vi "detect chassis modules.vi"(8 "error in":errorcluster, 11 "Controller in":refnum<class "Controller.lvclass">=refnum) -> (0 "error out":errorcluster, 3 "Controller out":refnum<class "Controller.lvclass">)   [LabVIEW 2013, in "SMI.lvlib" / "Chassis.lvclass"]
uses:
  Chassis.lvclass
  C Series Module/C Series Module.lvclass
  PXI Module/PXI Module.lvclass
  Controller/Controller.lvclass
  Device/Device.lvclass
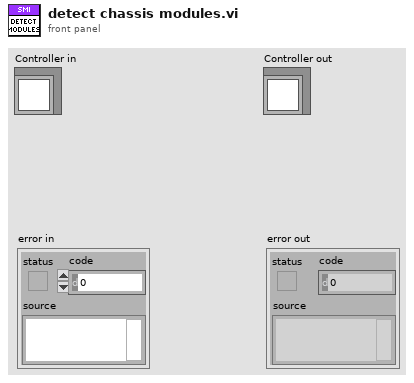
[diagram p1: front panel]
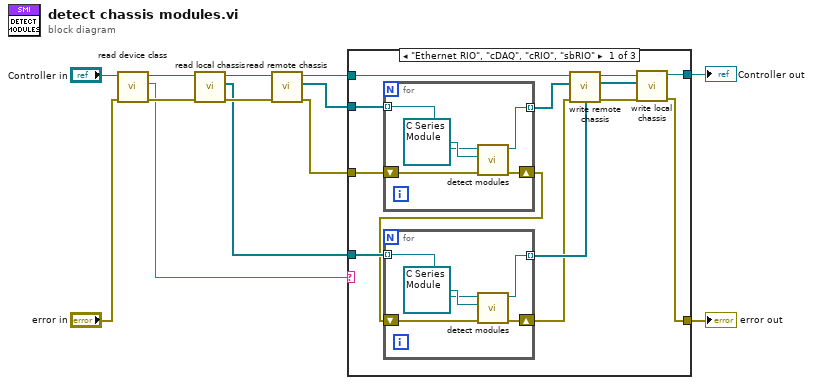
[diagram p0: block diagram]
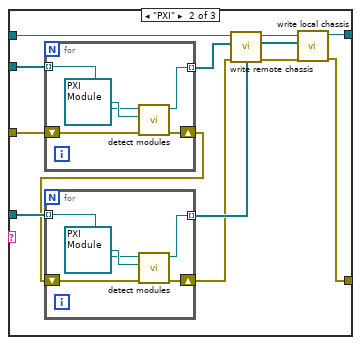
[diagram p2: hidden frame]
diagram:
  n1 = call-dynamic "read device class.vi"("error in"="error in", "device in"="Controller in") -> ("error out"=w9:errorcluster, "device class"=w1:string, "device out"=w2:refnum<class "Device.lvclass">)  [unwired: 7 in]
  n2 = call-dynamic "read local chassis.vi"("error in (no error)"=w9, "Controller in"=w2) -> ("error out"=w4:errorcluster, "local chassis"=w3:refnum<class "Chassis.lvclass">[], "Controller out"=w10:refnum<class "Controller.lvclass">)  [unwired: 7 in]
  n3 = call-dynamic "read remote chassis.vi"("error in (no error)"=w4, "Controller in"=w10) -> ("error out"=w8:errorcluster, "remote chassis"=w6:refnum<class "Chassis.lvclass">[], "Controller out"=w7:refnum<class "Controller.lvclass">)  [unwired: 7 in]
  n4 = case shown="\"Ethernet RIO\", \"cDAQ\", \"cRIO\", \"sbRIO\"" w1 {
    tunnel: [w14 w36 w59] -> w11
    tunnel: w8 -> [w18 w40 w59]
    tunnel: w3 -> [w25 w47 _]
    tunnel: w6 -> [w24 w46 _]
    tunnel: w7 -> [w23 w45 w58]
    tunnel: [w21 w43 w58] -> w5
    frame "Ethernet RIO", "cDAQ", "cRIO", "sbRIO" {
      n5 = for {
        tunnel: w24 -> [w29] mode=indexing
        tunnel: [w28] -> w20 mode=indexing
        shift-right: [w27] -> w17
        shift-left: w18 -> [w26]
        n6 = call-dynamic "detect modules.vi"("error in"=w26, "Module in"=refnum<class "C Series Module.lvclass"> refnum ("SMI.lvlib:C Series Module.lvclass"), "Chassis in"=w29) -> ("error out"=w27:errorcluster, "Chassis out"=w28:refnum<class "Chassis.lvclass">)  [unwired: 6 in, 1 out]
      }
      n7 = for {
        tunnel: w25 -> [w34] mode=indexing
        tunnel: [w33] -> w19 mode=indexing
        shift-right: [w32] -> w15
        shift-left: w17 -> [w31]
        n8 = call-dynamic "detect modules.vi"("error in"=w31, "Module in"=refnum<class "C Series Module.lvclass"> refnum ("SMI.lvlib:C Series Module.lvclass"), "Chassis in"=w34) -> ("error out"=w32:errorcluster, "Chassis out"=w33:refnum<class "Chassis.lvclass">)  [unwired: 6 in, 1 out]
      }
      n9 = call-dynamic "write remote chassis.vi"("error in (no error)"=w15, "remote chassis"=w20, "Controller in"=w23) -> ("error out"=w16:errorcluster, "Controller out"=w22:refnum<class "Controller.lvclass">)  [unwired: 7 in]
      n10 = call-dynamic "write local chassis.vi"("error in (no error)"=w16, "local chassis"=w19, "Controller in"=w22) -> ("error out"=w14:errorcluster, "Controller out"=w21:refnum<class "Controller.lvclass">)  [unwired: 7 in]
    }
    frame "PXI" {
      n11 = for {
        tunnel: w46 -> [w51] mode=indexing
        tunnel: [w50] -> w42 mode=indexing
        shift-right: [w49] -> w39
        shift-left: w40 -> [w48]
        n12 = call-dynamic "detect modules.vi"("error in"=w48, "PXI Module in"=refnum<class "PXI Module.lvclass"> refnum ("SMI.lvlib:PXI Module.lvclass"), "Chassis in"=w51) -> ("error out"=w49:errorcluster, "Chassis out"=w50:refnum<class "Chassis.lvclass">)  [unwired: 6 in, 1 out]
      }
      n13 = for {
        tunnel: w47 -> [w56] mode=indexing
        tunnel: [w55] -> w41 mode=indexing
        shift-right: [w54] -> w37
        shift-left: w39 -> [w53]
        n14 = call-dynamic "detect modules.vi"("error in"=w53, "PXI Module in"=refnum<class "PXI Module.lvclass"> refnum ("SMI.lvlib:PXI Module.lvclass"), "Chassis in"=w56) -> ("error out"=w54:errorcluster, "Chassis out"=w55:refnum<class "Chassis.lvclass">)  [unwired: 6 in, 1 out]
      }
      n15 = call-dynamic "write remote chassis.vi"("error in (no error)"=w37, "remote chassis"=w42, "Controller in"=w45) -> ("error out"=w38:errorcluster, "Controller out"=w44:refnum<class "Controller.lvclass">)  [unwired: 7 in]
      n16 = call-dynamic "write local chassis.vi"("error in (no error)"=w38, "local chassis"=w41, "Controller in"=w44) -> ("error out"=w36:errorcluster, "Controller out"=w43:refnum<class "Controller.lvclass">)  [unwired: 7 in]
    }
    frame Default {
    }
  }
  "error out" <- w11
  "Controller out" <- w5
